vi "Car Wash Main.vi"() -> ()   [LabVIEW 2016, in "CLD Exam - Car Wash.lvlib"]
uses:
  CLD Exam - Car Wash.lvlib
  Controls/Car Wash Indicators.ctl
  Controls/Wash Options.ctl
  <vilib>/Utility/sysdir.llb/System Directory Type.ctl
  Error/Classes/Error Interface/Dialog Types.ctl
  Classes/Assembler/Assembler.lvclass
  Error/Stream Error.lvlib
  Error/Classes/Error Interface/Error Interface.lvclass
panel:
  in  "Start":bool
  out "Elapsed Time":dbl format="%0.2f"
  in  "stop":bool
  out "Wash Entry":bool
  in  "Wash Options":T1
  in  "Car Position Slider":u8(slide) max=3 scale=0.0..4.0
  out "Car Wash Indicators":T2
  # "Entry Console"
  # "Car Wash Display"
  # "Car Position Simulation"
  # "Pre-Soak\nH-P Wash\nL-P Wax\nSpot Free Rinse"
  # "Underbody Wash\nBug Remover"
  # "Tire Shine\nAir Dry"
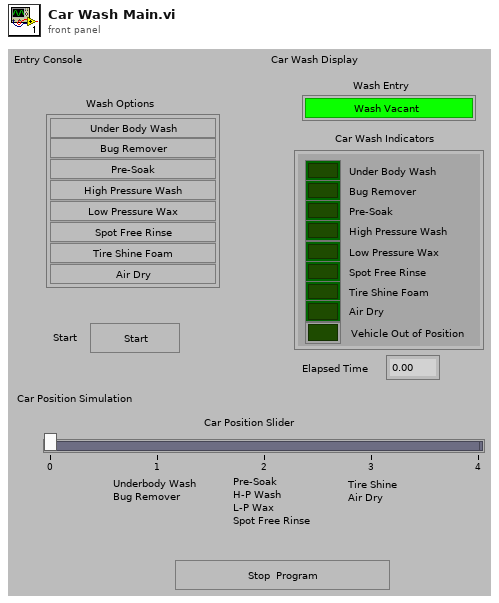
[diagram p1: front panel]
types:
  T1 = typedef "CLD Exam - Car Wash.lvlib/Wash Options.ctl" = cluster{"Underbody Wash":bool, "Bug Remover":bool, "Pre-Soak":bool, "High Pressure Wash":bool, "Low Pressure Wax":bool, "Spot Free Rinse":bool, "Tire Shine Foam":bool, "Air Dry":bool}
  T2 = typedef "CLD Exam - Car Wash.lvlib/Car Wash Indicators.ctl" = cluster{"Under Body Wash":bool, "Bug Remover":bool, "Pre-Soak":bool, "High Pressure Wash":bool, "Low Pressure Wax":bool, "Spot Free Rinse":bool, "Tire Shine Foam":bool, "Air Dry":bool, "Vehicle Out of Position":bool}
  T3 = typedef "Stream Error.lvlib/Error Interface.lvclass/Dialog Types.ctl" = enum16{"No Dialog", "Continue Dialog", "Stop Dialog", "Abort Dialog"}
  T4 = typedef "System Directory Type.ctl" = i32
  T5 = enum32{"invalid app kind", "Development System", "Run Time System", "Student Edition", "Embedded LabVIEW", "Evaluation", "Custom"}
  T6 = enum32{"Invalid", "Standard", "Closed", "Hidden", "Minimized", "Maximized"}
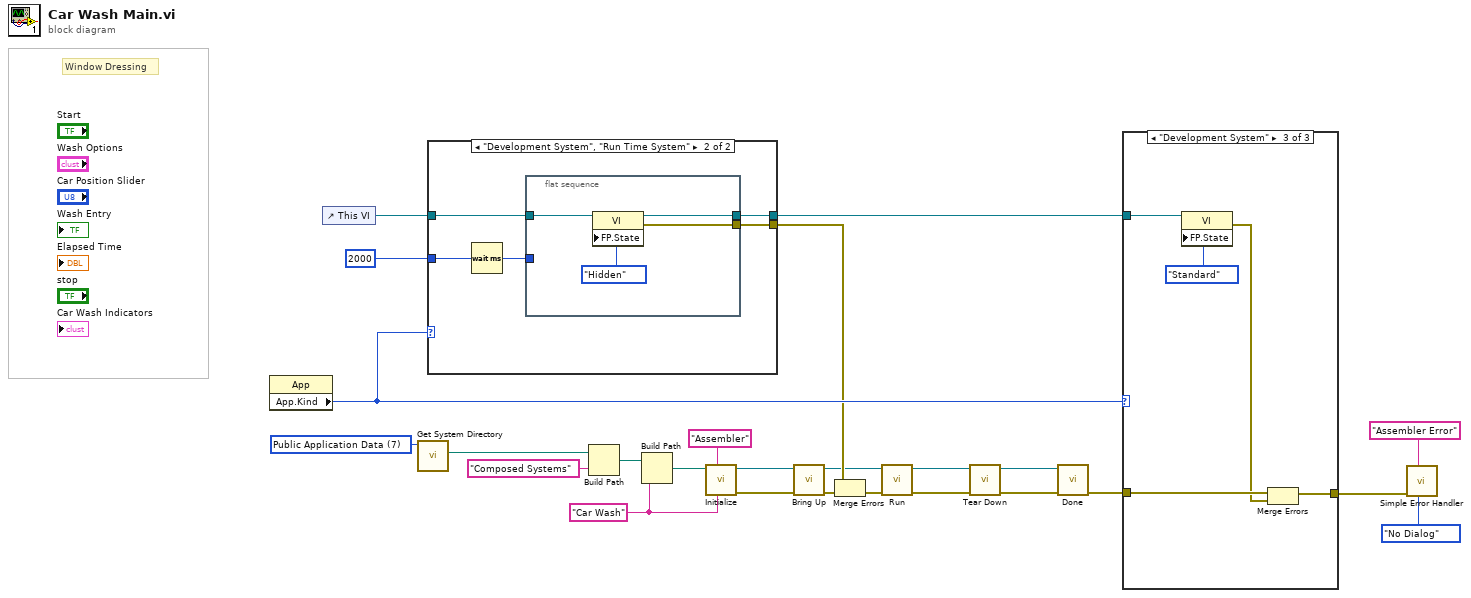
[diagram p0: block diagram]
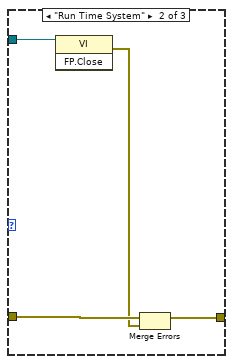
[diagram p3: hidden frame]
diagram:
  w23 = T4 7 items=["User Home"=0, "User Desktop"=1, "User Documents"=2, "User Application Data"=3, "User Preferences"=4, "User Temporary"=5, "Public Documents"=6, "Public Application Data"=7, "Public Preferences"=8, "Public Cache"=13, "System Core Libraries"=9, "System Installed Libraries"=10, "Application Files"=11, "Boot Volume Root"=12] ("system directory type")
  w5 = "Car Wash" ("iName")
  # "Window Dressing"
  n1 = property class="App"() -> ("App.Kind"=w19:T5)  [unwired: 2 in, 2 out]
  n2 = control-ref of="This VI"() -> (w20:refnum<vi>)
  n3 = call <vilib>:"Get System Directory.vi"("system directory type"=w23) -> ("system directory"=w22:path)  [unwired: 10 in]
  n4 = case shown="\"Development System\", \"Run Time System\"" w19 {
    tunnel: u32 2000 ("milliseconds to wait") -> [_ w31]
    tunnel: w20 -> [w26 w29]
    tunnel: [w26 w28] -> w18
    tunnel: [_ w27] -> w11
    frame Default {
    }
    frame "Development System", "Run Time System" {
      n5 = Wait (ms)(milliseconds to wait=w31) -> (millisecond timer value=w30:u32)
      n6 = flat-sequence {
        tunnel: w30 -> [_]
        tunnel: w29 -> [w35]
        tunnel: [w34] -> w28
        tunnel: [w33] -> w27
        frame #0 {
          n7 = property class="VI"(reference=w35, "FP.State"=T6."Hidden" ("Front Panel Window:State")) -> (reference out=w34:refnum<vi>, error out=w33:errorcluster)  [unwired: 1 in]
        }
      }
    }
  }
  n8 = Build Path(base path=w22, name or relative path="Composed Systems") -> (appended path=w24:path)
  n9 = Build Path(base path=w24, name or relative path=w5) -> (appended path=w4:path)
  n10 = call "Initialize.vi"("iName"=w5, "iType"="Assembler", "Application Data"=w4) -> ("error out"=w17:errorcluster, "Assembler out"=w10:refnum<class "Assembler.lvclass">)  [unwired: 7 in]
  n11 = call "Bring Up.vi"("error in (no error)"=w17, "Assembler in"=w10) -> ("error out"=w16:errorcluster, "Assembler out"=w9:refnum<class "Assembler.lvclass">)  [unwired: 8 in]
  n12 = Merge Errors(w11, w16) -> (w12:errorcluster)
  n13 = call "Run.vi"("error in (no error)"=w12, "Assembler in"=w9) -> ("error out"=w15:errorcluster, "Assembler out"=w8:refnum<class "Assembler.lvclass">)  [unwired: 8 in]
  n14 = call "Tear Down.vi"("error in (no error)"=w15, "Assembler in"=w8) -> ("error out"=w14:errorcluster, "Assembler out"=w7:refnum<class "Assembler.lvclass">)  [unwired: 8 in]
  n15 = call "Done.vi"("error in (no error)"=w14, "Assembler in"=w7) -> ("error out"=w13:errorcluster)  [unwired: 9 in]
  n16 = case shown="\"Development System\"" w19 {
    tunnel: w18 -> [_ w40 w45]
    tunnel: w13 -> [w36 w39 w44]
    tunnel: [w36 w37 w42] -> w3
    frame Default {
    }
    frame "Run Time System" {
      n17 = invoke class="VI" method="FP.Close"(reference=w40) -> (error out=w38:errorcluster)  [unwired: 2 in, 2 out]
      n18 = Merge Errors(w39, w38) -> (w37:errorcluster)
    }
    frame "Development System" {
      n19 = property class="VI"(reference=w45, "FP.State"=T6."Standard" ("Front Panel Window:State")) -> (error out=w43:errorcluster)  [unwired: 1 in, 1 out]
      n20 = Merge Errors(w44, w43) -> (w42:errorcluster)
    }
  }
  n21 = call "Simple Error Handler.vi"("Dialog Type"=Dialog_Types."No Dialog", "Window Title"="Assembler Error", "Error In"=w3) -> ()  [unwired: 7 in, 2 out]
